vi "Untitled 3.vi"() -> ()   [LabVIEW 2014]
uses:
  controls/Control ConfigurationSam.ctl
panel:
  in  "Append":bool
  in  "Stop Button":bool
  out "appended array 2":dbl[](array[numeric])
  out "appended array":dbl[](array[numeric])
  out "initialized array":T1[](array[typedef])
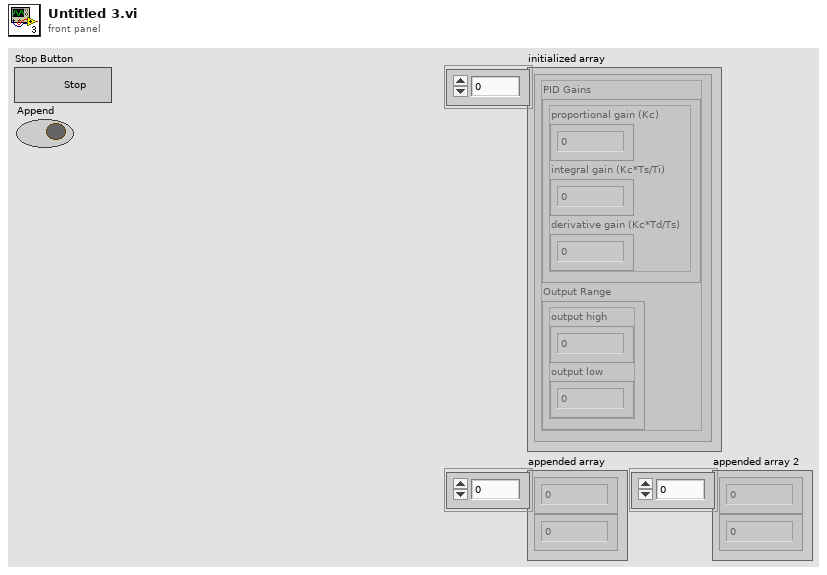
[diagram p1: front panel]
types:
  T1 = typedef "Control ConfigurationSam.ctl" = cluster{"PID Gains":cluster{"proportional gain (Kc)":dbl, "integral gain (Kc*Ts/Ti)":dbl, "derivative gain (Kc*Td/Ts)":dbl}, "Output Range":cluster{"output high":dbl, "output low":dbl}}
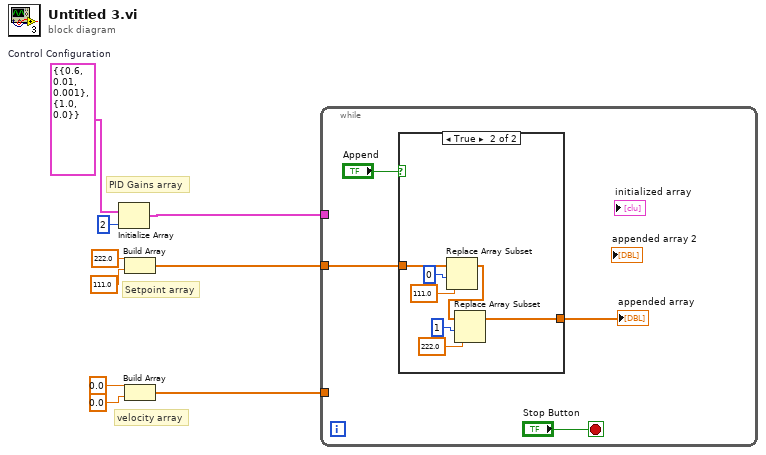
[diagram p0: block diagram]
diagram:
  w9 = T1 {"PID Gains"={"proportional gain (Kc)"=0.6, "integral gain (Kc*Ts/Ti)"=0.01, "derivative gain (Kc*Td/Ts)"=0.001}, "Output Range"={"output high"=1.0, "output low"=0.0}}  # Control Configuration
  # "velocity array"
  # "PID Gains array"
  # "Setpoint array"
  n1 = Initialize Array(w9, 2 ("dimension size")) -> (w3:T1[])
  n2 = Build Array(222.0, 111.0) -> (w2:dbl[])
  n3 = Build Array(0.0, 0.0) -> (w1:dbl[])
  n4 = while {
    tunnel: w3 -> [_]
    tunnel: w2 -> [w11]
    tunnel: w1 -> [_]
    stop <- "Stop Button" stop-if-true
    n5 = case shown="True" "Append" {
      tunnel: w11 -> [w14 w17]
      tunnel: [w14 w15] -> w10
      frame False {
      }
      frame True {
        n6 = Replace Array Subset(array=w17, new element=111.0 ("new element/subarray"), index=0) -> (w16:dbl[])
        n7 = Replace Array Subset(array=w16, new element=222.0 ("new element/subarray"), index=1) -> (w15:dbl[])
      }
    }
    "appended array" <- w10
  }
